vi "check memory limit.vi"(8 "error in (no error)":errorcluster caption="에러 입력(에러 없음)", 10 "bytes of waveform":i32[](array[numeric]), 11 "Haptic IC 입력":refnum<class "Haptic IC.lvclass">) -> (0 "error out":errorcluster caption="에러 출력", 1 "message":string, 2 "disable?":T1(ring), 3 "Haptic IC 출력":refnum<class "Haptic IC.lvclass">)   [LabVIEW 2020, in "Haptic IC.lvclass"]
uses:
  Haptic IC.lvclass
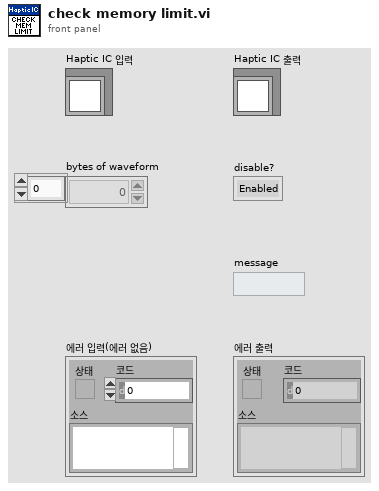
[diagram p1: front panel]
types:
  T1 = enum8{"Enabled", "Disabled", "Disabled and Grayed Out"}
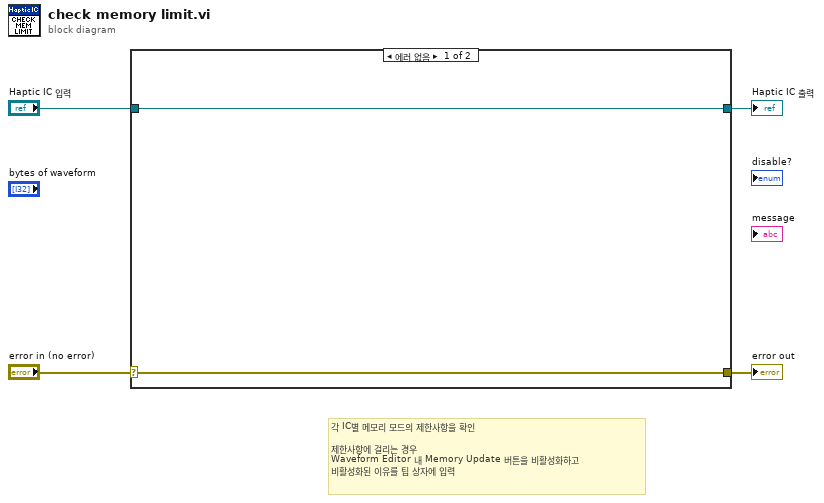
[diagram p0: block diagram]
diagram:
  # "각 IC별 메모리 모드의 제한사항을 확인\n\n제한사항에 걸리는 경우 \nWaveform Editor 내 Memory Update 버튼을 비활성화하고\n비활성화된 이유를 팁 상자에 입력"
  n1 = case shown="에러 없음" "error in (no error)" {
    selector: "error in (no error)" -> [w5 w8]
    tunnel: [w5 w8] -> w3
    tunnel: [w6 w7] -> w1
    tunnel: "Haptic IC 입력" -> [w6 w7]
    frame No Error {
    }
    frame Error {
    }
  }
  "error out" <- w3
  "Haptic IC 출력" <- w1
